vi "blokada wysylania jazda.vi"(6 "wysylanie":bool, 10 "X axis":i32, 11 "Y axis":i32) -> (0 "fall edge wysl":bool, 1 "blokada jazdy":bool, 3 "zakresy":cluster{"zak2":bool, "zak1":bool})   [LabVIEW 2015]
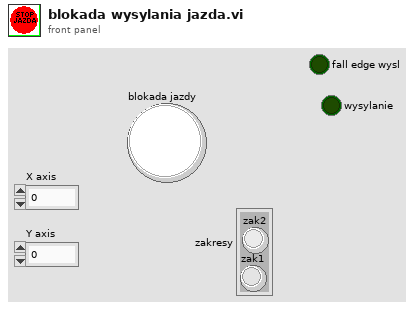
[diagram p1: front panel]
types:
  T1 = enum16{"Rising Edge", "Falling Edge", "Any Edge"}
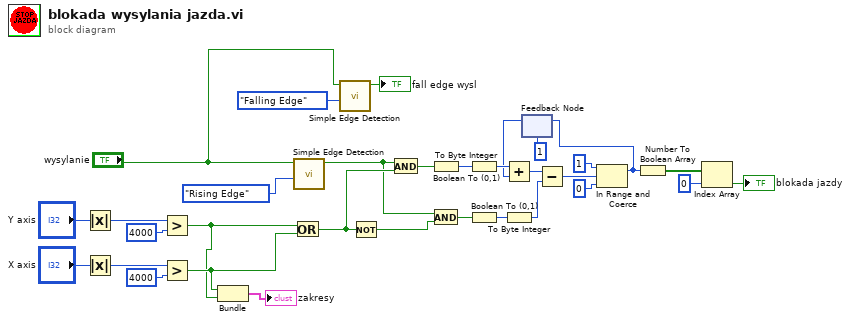
[diagram p0: block diagram]
diagram:
  n1 = Absolute Value(x="Y axis") -> (abs(x)=w25:i32)
  n2 = Absolute Value(x="X axis") -> (abs(x)=w28:i32)
  n3 = Greater?(x=w25, y=4000) -> (0:w3:bool)
  n4 = Greater?(x=w28, y=4000) -> (0:w4:bool)
  n5 = Bundle(w4, w3) -> (→"zakresy":cluster{bool, bool})  [unwired: 1 in]
  n6 = Or(x=w3, y=w4) -> (x .or. y?=w32:bool)
  n7 = call "Simple Edge Detection.vi"("Mode"=T1."Rising Edge", "clk_in"="wysylanie") -> ("edge?"=w9:bool)  [unwired: 9 in]
  n8 = call "Simple Edge Detection.vi"("Mode"=T1."Falling Edge", "clk_in"="wysylanie") -> ("edge?"=→"fall edge wysl":bool)  [unwired: 9 in]
  n9 = Not(x=w32) -> (.not. x?=w31:bool)
  n10 = And(x=w9, y=w32) -> (x .and. y?=w23:bool)
  n11 = Boolean To (0,1)(Boolean=w23) -> (0, 1=w15:i16)
  n12 = And(x=w9, y=w31) -> (x .and. y?=w24:bool)
  n13 = To Byte Integer(number=w15) -> (8bit integer=w14:i8)
  n14 = Boolean To (0,1)(Boolean=w24) -> (0, 1=w13:i16)
  n15 = To Byte Integer(number=w13) -> (8bit integer=w12:i8)
  n16 = feedback #1(i8 1 ("lower limit")) -> (w10:i8)
  n17 = Add(x=w14, y=w10) -> (x+y=w22:i8)
  n18 = Subtract(x=w22, y=w12) -> (x-y=w21:i8)
  n19 = In Range and Coerce(upper limit=i8 1 ("lower limit"), x=w21, lower limit=i8 0) -> (coerced(x)=w11:i8)  [unwired: 1 out]
  n20 = feedback-in #1(w11) -> ()
  n21 = Number To Boolean Array(number=w11) -> (Boolean array=w17:bool[])
  n22 = Index Array(array=w17, index=0) -> (element=→"blokada jazdy":bool)
